vi "Connect.vi"(8 "error in (no error)":errorcluster, 11 "modbus in":refnum<class "libmodbus.lvclass">) -> (0 "error out":errorcluster, 3 "modbus out":refnum<class "libmodbus.lvclass">)   [LabVIEW 2017, in "libmodbus.lvlib" / "libmodbus.lvclass"]
doc: "Generates an error from the actual errno."
uses:
  libmodbus.lvclass
  libmodbus.lvclass/libmodbus.ctl
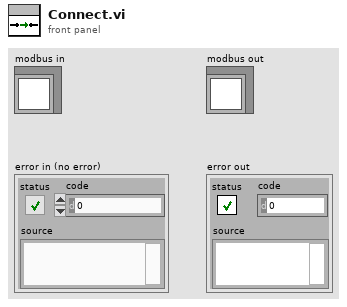
[diagram p1: front panel]
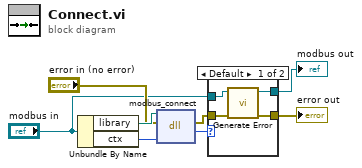
[diagram p0: block diagram]
diagram:
  n1 = Unbundle By Name("modbus in") -> ("library"=w7:path, "ctx"=w8:i64)
  n2 = dll-call lib="?" fn="modbus_connect"(path in=w7, error in="error in (no error)", "ctx"=w8) -> (error out=w3:errorcluster, "int"=w5:i32)  [unwired: 2 in, 1 out]
  n3 = case shown="Default" w5 {
    tunnel: [w11 w14] -> w4
    tunnel: w3 -> [w12 w14]
    tunnel: "modbus in" -> [w10 w13]
    tunnel: [w9 w13] -> w1
    frame Default {
      n4 = call "Generate Error.vi"("error in (no error)"=w12, "modbus in"=w10) -> ("error out"=w11:errorcluster, "modbus out"=w9:refnum<class "libmodbus.lvclass">)  [unwired: 8 in]
    }
    frame 0 {
    }
  }
  "modbus out" <- w1
  "error out" <- w4
